vi "teste do estimador de velocidade.vi"() -> ()   [LabVIEW 2016]
uses:
  SSL Detection Frame.ctl
  SSL Detection Robot.ctl
  SSL Detection Ball.ctl
  <vilib>/Utility/tcp.llb/UDP Multicast Read-Only Open.vi
panel:
  out "w (rad/s)":dbl
  out "V_y\n(cm/s)":dbl(knob) scale=0.0..10.0
  out "V_x (cm/s)":dbl(knob) scale=0.0..10.0
  out "error out":errorcluster
  out "Detection Frame Out":T1
  in  "stop":bool
  in  "camera_id":u32
  out "LAST DATA":T4
  in  "life time":dbl=1.0 format="%#_13g"
  in  "port":u16
  in  "String":string
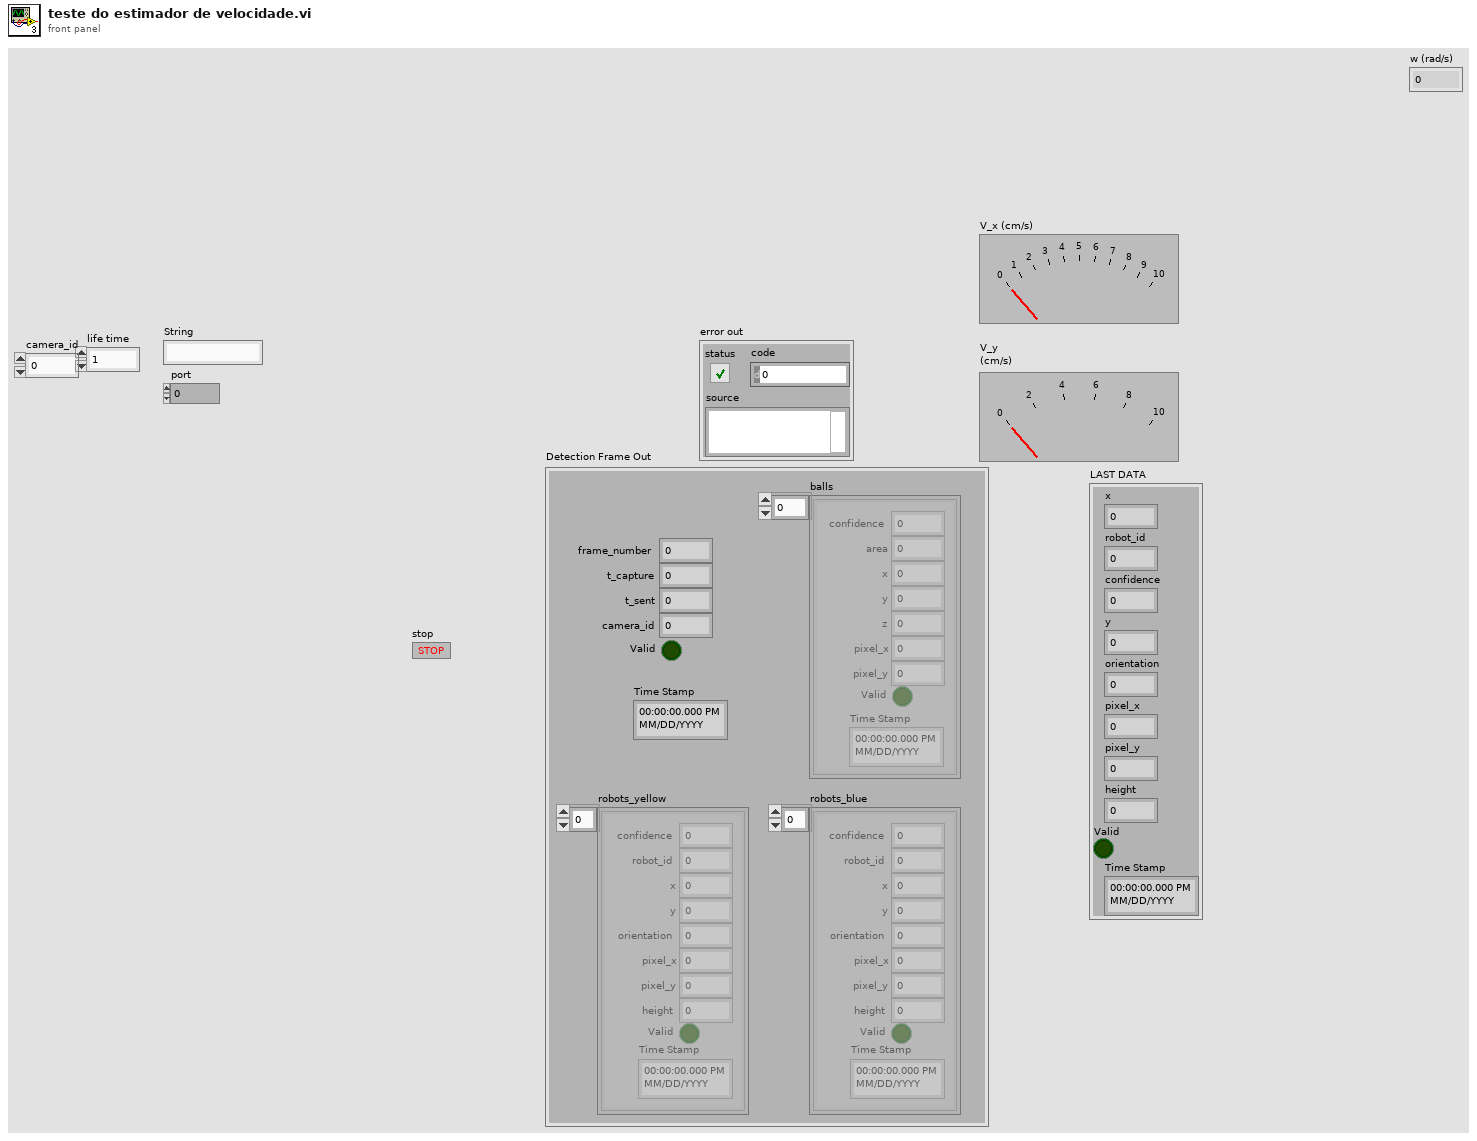
[diagram p1: front panel]
types:
  T1 = typedef "SSL Detection Frame.ctl" = cluster{"frame_number":u32, "t_capture":dbl, "t_sent":dbl, "camera_id":u32, "robots_yellow":T2[], "robots_blue":T2[], "balls":T3[], "Valid":bool, "Time Stamp":timestamp}
  T2 = typedef "SSL Detection Robot.ctl" = cluster{"x":dbl, "robot_id":u32, "confidence":sgl, "y":sgl, "orientation":sgl, "pixel_x":sgl, "pixel_y":sgl, "height":sgl, "Valid":bool, "Time Stamp":timestamp}
  T3 = typedef "SSL Detection Ball.ctl" = cluster{"x":sgl, "area":u32, "confidence":sgl, "y":sgl, "z":sgl, "pixel_x":sgl, "pixel_y":sgl, "Valid":bool, "Time Stamp":timestamp}
  T4 = cluster{"x":dbl, "robot_id":u32, "confidence":sgl, "y":sgl, "orientation":sgl, "pixel_x":sgl, "pixel_y":sgl, "height":sgl, "Valid":bool, "Time Stamp":timestamp}
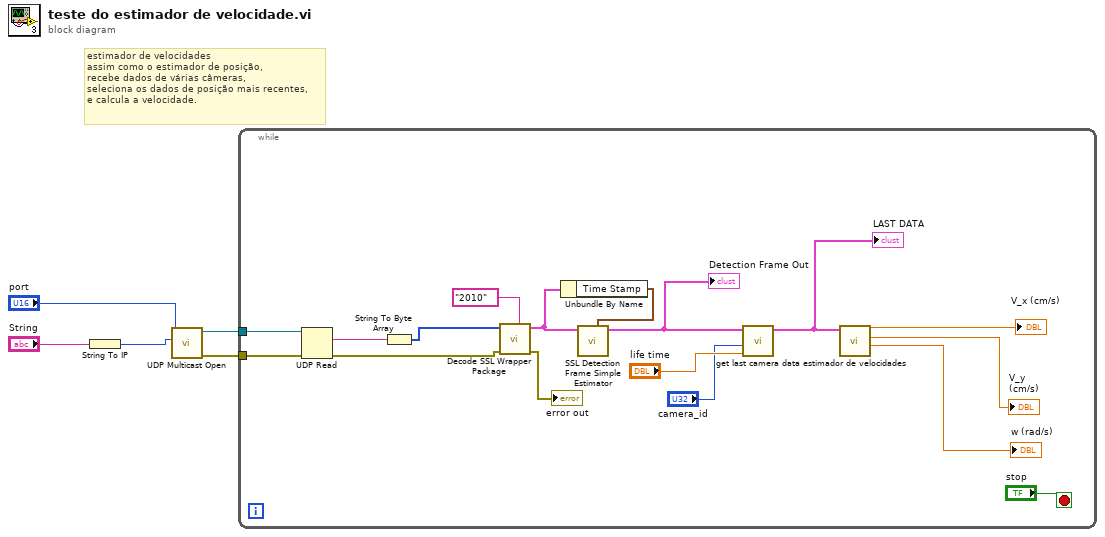
[diagram p0: block diagram]
diagram:
  # "estimador de velocidades\nassim como o estimador de posição,\nrecebe dados de várias câmeras,\nseleciona os dados de posição mais recentes,\ne calcula a velocidade."
  n1 = String To IP(1:"String") -> (0:w4:u32)
  n2 = call-poly <vilib>:"UDP Multicast Open.vi"("multicast addr"=w4, "port"="port") -> ("error out"=w1:errorcluster, "connection ID"=w2:refnum<k16>)  [unwired: 7 in, 1 out]
  n3 = while {
    tunnel: w2 -> [w22]
    tunnel: w1 -> [w21]
    stop <- "stop" stop-if-true
    n4 = UDP Read(connection ID=w22, 8:w21) -> (data out=w20:string, error out=w18:errorcluster)  [unwired: 2 in, 3 out]
    n5 = String To Byte Array(string=w20) -> (unsigned byte array=w19:u8[])
    n6 = call "Decode SSL Wrapper Package.vi"("Version"="2010", "error in (no error)"=w18, "unsigned byte array"=w19) -> ("error out"=→"error out":errorcluster, "Detection Frame"=w15:T1)  [unwired: 5 in, 2 out]
    n7 = Unbundle By Name(w15) -> ("Time Stamp"=w14:timestamp)
    n8 = call "SSL Detection Frame Simple Estimator.vi"("Now"=w14, "Detection Frame In"=w15) -> ("Detection Frame Out"=w10:T1)  [unwired: 9 in]
    "Detection Frame Out" <- w10
    n9 = call "get last camera data.vi"("life time"="life time", "camera_id"="camera_id", "Detection Frame In"=w10) -> ("pos estimation"=w6:T2)  [unwired: 8 in]
    "LAST DATA" <- w6
    n10 = call "estimador de velocidades.vi"("estimation"=w6) -> ("angular speed (rad/s)"=→"w (rad/s)":dbl, "speed (cm/s)"=→"V_y\n(cm/s)":dbl, "speed (cm/s) 2"=→"V_x (cm/s)":dbl)  [unwired: 8 in]
  }
